vi "getSubnetData.vi"(11 "Subnet in":refnum<class "Subnet.lvclass">) -> (2 "SubnetData":T1, 3 "Subnet out":refnum<class "Subnet.lvclass">)   [LabVIEW 2016, in "Subnet.lvclass"]
uses:
  Subnet.lvclass
  DataTypes/SubnetData.ctl
  Common_RT_Modbus/IModbus/IModbus.lvclass
  DataTypes/SubnetConstants.ctl
  Common_RT_HPILC/HPILC/HPILC.lvclass
  DataTypes/ILCIndexData.ctl
  DataTypes/ILCTypes.ctl
  Common_RT_MTILC/MTILC/MTILC.lvclass
  Common_RT_MDILC/MDILC/MDILC.lvclass
  Common_RT_MIILC/MIILC/MIILC.lvclass
  DataTypes/SubnetCommand.ctl
  DataTypes/SubnetTelemetry.ctl
  Subnet.lvclass/Subnet.ctl
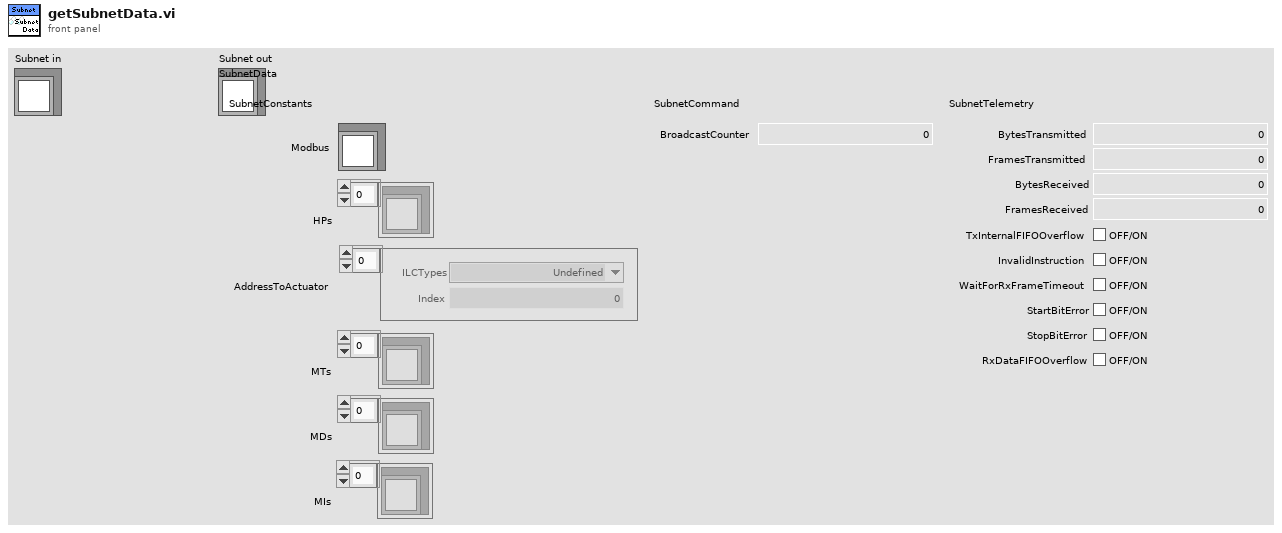
[diagram p1: front panel]
types:
  T1 = typedef "SubnetData.ctl" = cluster{"SubnetConstants":T2, "SubnetCommand":T5, "SubnetTelemetry":T6}
  T2 = typedef "SubnetConstants.ctl" = cluster{"Modbus":refnum<class "IModbus.lvclass">, "HPs":refnum<class "HPILC.lvclass">[], "AddressToActuator":T3[], "MTs":refnum<class "MTILC.lvclass">[], "MDs":refnum<class "MDILC.lvclass">[], "MIs":refnum<class "MIILC.lvclass">[]}
  T3 = typedef "ILCIndexData.ctl" = cluster{"ILCTypes":T4, "Index":i32}
  T4 = typedef "ILCTypes.ctl" = enum16{"Undefined", "SAA", "DAA", "HP", "MT", "MD", "MI"}
  T5 = typedef "SubnetCommand.ctl" = cluster{"BroadcastCounter":u8}
  T6 = typedef "SubnetTelemetry.ctl" = cluster{"BytesTransmitted":u32, "FramesTransmitted":u32, "BytesReceived":u32, "FramesReceived":u32, "TxInternalFIFOOverflow":bool, "InvalidInstruction":bool, "WaitForRxFrameTimeout":bool, "StartBitError":bool, "StopBitError":bool, "RxDataFIFOOverflow":bool}
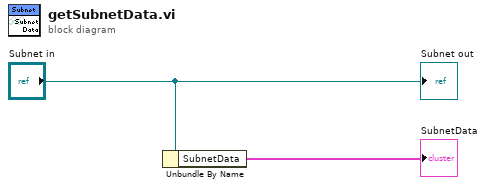
[diagram p0: block diagram]
diagram:
  n1 = Unbundle By Name("Subnet in") -> ("SubnetData"=→"SubnetData":T1)
  "Subnet out" <- "Subnet in"
